vi "Init Bfr Tx - UDP Connection.vi"(8 "error in (no error)":errorcluster, 11 "Tx Loop Data in":T1 {"Data Buffer" format="%016x"}) -> (0 "error out":errorcluster, 3 "Tx Loop Data out":T1 {"Data Buffer" format="%016x"})   [LabVIEW 2016, in "UDP-Custom-Device Engine.lvlib"]
uses:
  UDP-Custom-Device Engine.lvlib
  Types/Engine - Buffered Tx Loop Data.ctl
  Shared/Types/Shared - Header Details.ctl
  Shared/Types/Shared - Buffered.PacketInfo.ctl
  <vilib>/NI/NIVS Inline Async API/_Data Access Engine/Data Access Engine/Types/ReadWrite.DVR.ctl
  <vilib>/NI/NIVS Inline Async API/_Data Access Engine/Access Type Classes/ReadWrite/ReadWrite.lvclass
  <vilib>/NI/NIVS Inline Async API/_Data Access Engine/Data Access Engine/Types/Read.DVR.ctl
  <vilib>/NI/NIVS Inline Async API/_Data Access Engine/Access Type Classes/Read/Read.lvclass
  <vilib>/NI/NIVS Inline Async API/_Data Access Engine/Data Access Engine/Types/Write.DVR.ctl
  <vilib>/NI/NIVS Inline Async API/_Data Access Engine/Access Type Classes/Write/Write.lvclass
  Shared/Types/Shared - Duplex Settings.ctl
  <vilib>/Utility/tcp.llb/UDP Multicast Write-Only Open.vi
  Shared/UDP-Custom-Device Shared.lvlib
  <vilib>/NI/NIVS Inline Async API/_Data Access Engine/Data Access Engine/Data Access Engine.lvclass
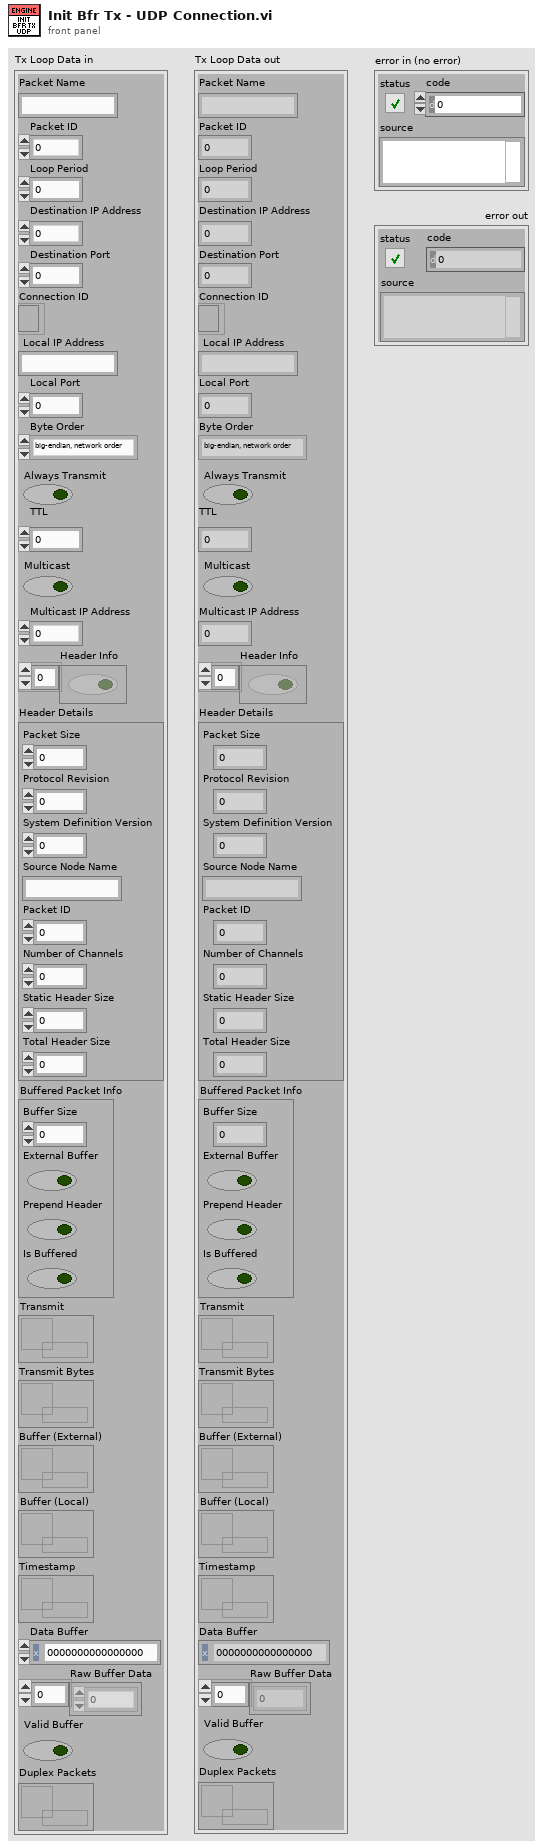
[diagram p1: front panel]
types:
  T1 = typedef "UDP-Custom-Device Engine.lvlib/Engine - Buffered Tx Loop Data.ctl" = cluster{"Packet Name":string, "Packet ID":i32, "Loop Period":u32, "Destination IP Address":u32, "Destination Port":u16, "Connection ID":refnum<k16>, "Local IP Address":string, "Local Port":i32, "Byte Order":enum16{"big-endian, network order", "native, host order", "little-endian"}, "Always Transmit":bool, "TTL":u16, "Multicast":bool, "Multicast IP Address":u32, "Header Info":bool[], "Header Details":T2, "Buffered Packet Info":T3, "Transmit":T4, "Transmit Bytes":T5, "Buffer (External)":T5, "Buffer (Local)":T6, "Timestamp":T5, "Data Buffer":u64, "Raw Buffer Data":u8[], "Valid Buffer":bool, "Duplex Packets":refnum<data-value>}
  T2 = typedef "UDP-Custom-Device Shared.lvlib/Shared - Header Details.ctl" = cluster{"Packet Size":u16, "Protocol Revision":u8, "System Definition Version":u64, "Source Node Name":string, "Packet ID":u32, "Number of Channels":u32, "Static Header Size":u16, "Total Header Size":u16}
  T3 = typedef "UDP-Custom-Device Shared.lvlib/Shared - Buffered.PacketInfo.ctl" = cluster{"Buffer Size":i32, "External Buffer":bool, "Prepend Header":bool, "Is Buffered":bool}
  T4 = typedef "Data Access Engine.lvlib/Data Access Engine.lvclass/ReadWrite.DVR.ctl" = refnum<data-value>
  T5 = typedef "Data Access Engine.lvlib/Data Access Engine.lvclass/Read.DVR.ctl" = refnum<data-value>
  T6 = typedef "Data Access Engine.lvlib/Data Access Engine.lvclass/Write.DVR.ctl" = refnum<data-value>
  T7 = typedef "UDP-Custom-Device Shared.lvlib/Shared - Duplex Settings.ctl" = cluster{"Transmit Packet ID":i32, "Receive Packet ID":i32, "Multicast":bool, "Multicast Address":string, "IP Address":string, "Port":u16, "TTL":u16, "Duplex Connection":refnum<k16>}
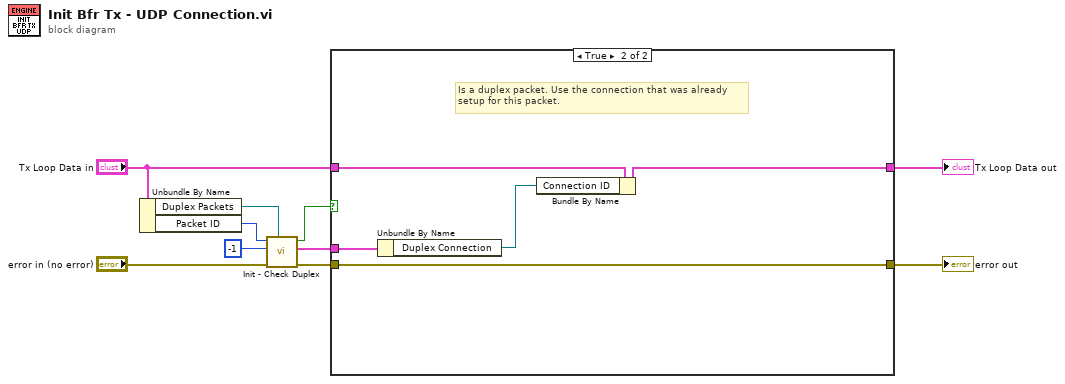
[diagram p0: block diagram]
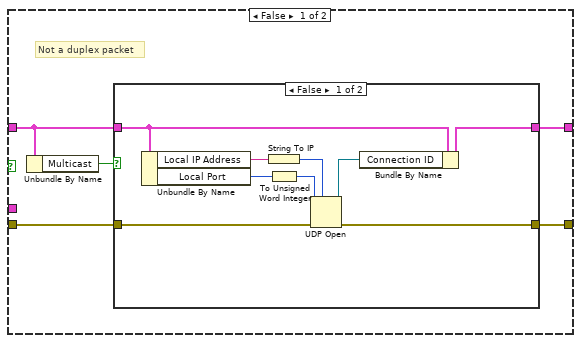
[diagram p2: hidden frame]
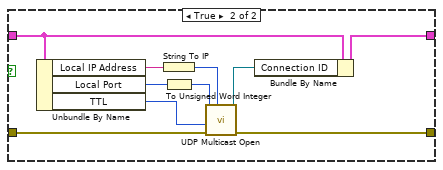
[diagram p3: hidden frame]
diagram:
  n1 = Unbundle By Name("Tx Loop Data in") -> ("Duplex Packets"=w8:refnum<data-value>, "Packet ID"=w5:i32)
  n2 = call "Init - Check Duplex.vi"("Duplex Packets"=w8, "error in (no error)"="error in (no error)", "Receive Packet ID"=-1, "Transmit Packet ID"=w5) -> ("error out"=w3:errorcluster, "Duplex Settings"=w2:T7, "Is Duplex?"=w6:bool)  [unwired: 5 in]
  n3 = case shown="True" w6 {
    tunnel: w3 -> [w15 w35]
    tunnel: [w14 w35] -> w10
    tunnel: [w13 w37] -> w9
    tunnel: "Tx Loop Data in" -> [w12 w38]
    tunnel: w2 -> [_ w36]
    frame False {
      # "Not a duplex packet"
      n4 = Unbundle By Name(w12) -> ("Multicast"=w11:bool)
      n5 = case shown="False" w11 {
        tunnel: w15 -> [w19 w29]
        tunnel: [w18 w28] -> w14
        tunnel: w12 -> [w17 w27]
        tunnel: [w16 w26] -> w13
        frame False {
          n6 = Unbundle By Name(w17) -> ("Local IP Address"=w21:string, "Local Port"=w24:i32)
          n7 = String To IP(1:w21) -> (0:w20:u32)
          n8 = To Unsigned Word Integer(number=w24) -> (unsigned 16bit integer=w22:u16)
          n9 = UDP Open(7:w20, 8:w19, 11:w22) -> (port=w23:refnum<k16>, 0:w18:errorcluster)  [unwired: 2 in, 1 out]
          n10 = Bundle By Name(cluster=w17, "Connection ID"=w23) -> (w16:T1)
        }
        frame True {
          n11 = Unbundle By Name(w27) -> ("Local IP Address"=w31:string, "Local Port"=w34:i32, "TTL"=w25:u16)
          n12 = String To IP(1:w31) -> (0:w30:u32)
          n13 = To Unsigned Word Integer(number=w34) -> (unsigned 16bit integer=w32:u16)
          n14 = call-poly <vilib>:"UDP Multicast Open.vi"("net address"=w30, "error in (no error)"=w29, "time-to-live (1)"=w25, "port"=w32) -> ("error out"=w28:errorcluster, "connection ID"=w33:refnum<k16>)  [unwired: 6 in]
          n15 = Bundle By Name(cluster=w27, "Connection ID"=w33) -> (w26:T1)
        }
      }
    }
    frame True {
      # "Is a duplex packet. Use the connection that was already\nsetup for this packet."
      n16 = Unbundle By Name(w36) -> ("Duplex Connection"=w39:refnum<k16>)
      n17 = Bundle By Name(cluster=w38, "Connection ID"=w39) -> (w37:T1)
    }
  }
  "Tx Loop Data out" <- w9
  "error out" <- w10
